vi "User Info Message Callback.vi"(7 "Owner":refnum<class>, 11 "Message":refnum<class "Message.lvclass">) -> (0 "error out":errorcluster)   [LabVIEW 2020, in "LV Chat Server.lvclass"]
uses:
  LV Chat Server.lvclass
  <vilib>/IlluminatedG/lv-msg-simple/Stream-Simple-Msg/Message/Message.lvclass
  Data Types/User Info.ctl
  LV Chat Server.lvclass/LV Chat Server.ctl
  Data Types/Message ID.ctl
  8b6985b5-31a4-4f8f-9d19-d109e1dac7ef.vi
  6ee463a9-6330-4a6d-9728-e0f9e692d2e6.vi
  ddd42a80-e0b0-4c60-b3e6-7a086e111a44.vi
  ddd42a80-e0b0-4c60-b3e6-7a086e111a44.vi/cd1d5f5c-70bb-4037-9238-b7596cc892a6.vi
  ddd42a80-e0b0-4c60-b3e6-7a086e111a44.vi/054d6784-ec16-41ee-85a9-d07961f40e21.vi
  <vilib>/IlluminatedG/lv-msg-simple/Stream-Simple-Msg/Message/Get Data.vi
  <vilib>/IlluminatedG/lv-msg-simple/Stream-Simple-Msg/Message/_Create.vi
  <vilib>/IlluminatedG/lv-msg-simple/Stream-Simple-Msg/Message/Get Flattened Message.vi
  <vilib>/IlluminatedG/lv-msg-simple/Stream-Simple-Msg/Endpoint/Get Stream.vi
  <vilib>/IlluminatedG/lv-stream/stream/Stream.lvclass
  <vilib>/IlluminatedG/lv-msg-simple/Stream-Simple-Msg/Endpoint/Endpoint.lvclass
  <vilib>/IlluminatedG/lv-stream/URI/URI.lvclass
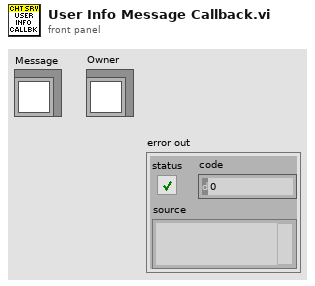
[diagram p1: front panel]
types:
  T1 = typedef "User Info.ctl" = cluster{"Name":string}
  T2 = typedef "Message ID.ctl" = enum16{"UserInfo", "UserList", "Message", "Disconnect"}
  T3 = typedef "LV Chat Server.lvclass/Ref Data.ctl" = cluster{"Endpoint Map":map{string, T4}, "User Map":map{string, string}}
  T4 = typedef "LV Chat Server.lvclass/User.ctl" = cluster{"Name":string, "IP":string, "Connected At":dbl, "Endpoint":refnum<class "Endpoint.lvclass">}
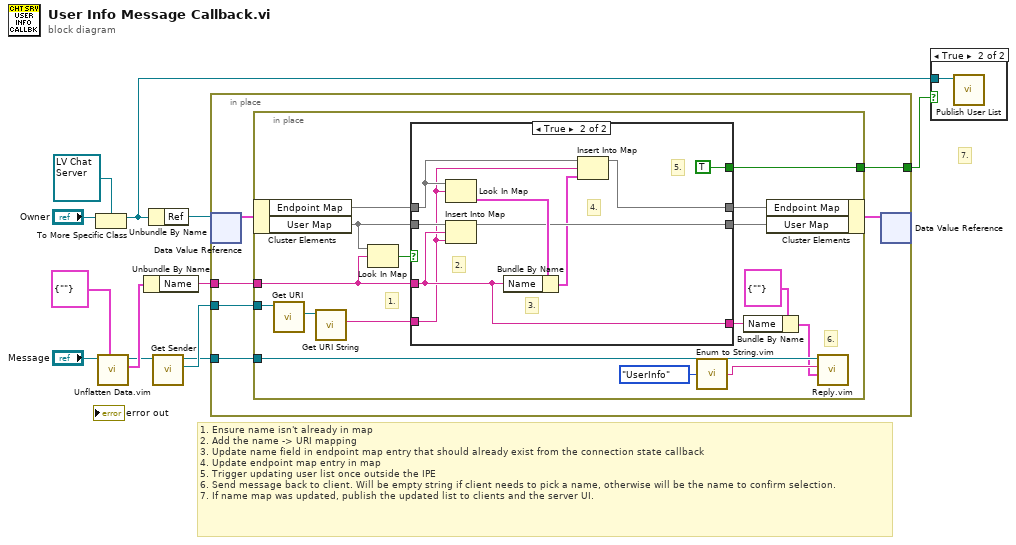
[diagram p0: block diagram]
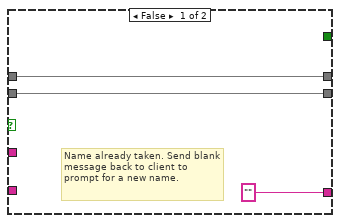
[diagram p3: hidden frame]
diagram:
  # "7."
  # "1. Ensure name isn't already in map\n2. Add the name -> URI mapping\n3. Update name field in endpoint map entry that should already exist from the connection state callback\n4. Update endpoint map entry in map\n5. Trigger updating user list once outside the IPE\n6. Send message back to client. Will be empty string if client needs to pick a name, otherwise will be the name to confirm selection.\n7. If name map was updated, publish the updated list to clients and the server UI."
  n1 = To More Specific Class(target class=refnum<class "LV Chat Server.lvclass"> refnum ("LV Chat Server.lvclass"), reference="Owner") -> (specific class reference=w1:refnum<class "LV Chat Server.lvclass">)  [unwired: 1 in, 1 out]
  n2 = call "Unflatten Data.vim"("Data Type"=T1 {"Name"=""} ("User Info"), "Message in"="Message") -> ("Unflattened Data"=w10:T1, "Message out"=w9:refnum<class "Message.lvclass">)  [unwired: 7 in, 1 out]
  n3 = Unbundle By Name(w10) -> ("Name"=w5:string)
  n4 = Unbundle By Name(w1) -> ("Ref"=w6:refnum<data-value>)
  n5 = call <vilib>:"Get Sender.vi"("Message in"=w9) -> ("Sender"=w4:refnum<class "Endpoint.lvclass">, "Message out"=w3:refnum<class "Message.lvclass">)  [unwired: 8 in, 1 out]
  n6 = in-place {
    in-place-border: w5 -> [w18]
    in-place-border: w4 -> [w15]
    in-place-border: w3 -> [w14]
    in-place-border: [w13] -> w2
    n7 = in-place-dvr #1(w6) -> (w17:T3)  [unwired: 1 out]
    n8 = in-place {
      in-place-border: w18 -> [w26]
      in-place-border: w15 -> [w33]
      in-place-border: w14 -> [w22]
      in-place-border: [w25] -> w13
      # "6."
      # "1."
      n9 = in-place-cluster #2(w17) -> ("Endpoint Map"=w28:map{string, T4}, "User Map"=w30:map{string, string})
      n10 = call <vilib>:"Get URI.vi"("Endpoint in"=w33) -> ("URI"=w32:refnum<class "URI.lvclass">)  [unwired: 8 in, 2 out]
      n11 = call <vilib>:"Get URI String.vi"("URI in"=w32) -> ("URI String"=w31:string)  [unwired: 8 in, 2 out]
      n12 = Look In Map(map=w30, key=w26) -> (key not found?=w34:bool)  [unwired: 1 in, 1 out]
      n13 = case shown="True" w34 {
        tunnel: w31 -> [_ w38]
        tunnel: w30 -> [w36 w46]
        tunnel: [w37 w41] -> w29
        tunnel: w28 -> [w37 w43]
        tunnel: [w36 w44] -> w27
        tunnel: w26 -> [_ w39]
        tunnel: [_ TRUE] -> w25
        tunnel: ["" w39] -> w20
        frame False {
          # "Name already taken. Send blank message back to client to prompt for a new name."
        }
        frame True {
          # "5."
          # "4."
          # "3."
          # "2."
          n14 = Look In Map(map=w43, key=w38) -> (value=w45:T4)  [unwired: 1 in, 1 out]
          n15 = Insert Into Map(map in=w46, key=w39, value=w38) -> (map out=w44:map{string, string})  [unwired: 2 out]
          n16 = Bundle By Name(cluster=w45, "Name"=w39) -> (w42:T4)
          n17 = Insert Into Map(map in=w43, key=w38, value=w42) -> (map out=w41:map{string, T4})  [unwired: 2 out]
        }
      }
      n18 = call "Enum to String.vim"("Enum"=Message_ID."UserInfo" ("Message ID")) -> ("Enum String"=w24:string)
      n19 = Bundle By Name(cluster=T1 {"Name"=""} ("User Info"), "Name"=w20) -> (w19:T1)
      n20 = in-place-cluster #2("Endpoint Map"=w29, "User Map"=w27) -> (w16:T3)
      n21 = call "Reply.vim"("Reply Data (With ID String)"=w19, "Reply Message (Or ID String)"=w24, "Message in"=w22) -> ()  [unwired: 7 in, 2 out]
    }
    n22 = in-place-dvr #1(w16) -> ()  [unwired: 2 out]
  }
  n23 = case shown="True" w2 {
    tunnel: w1 -> [_ w47]
    frame False {
    }
    frame True {
      n24 = call "Publish User List.vi"("LV Chat Server in"=w47) -> ()  [unwired: 9 in, 2 out]
    }
  }
